vi "MB Ethernet Master Query.vi"(4 "Timeout":i32=5000, 6 "MBAP Header":cluster{"Transaction ID":u16, "Unit ID":u8}, 7 "Modbus Data Unit In":T2={"Function Code"=1, "Data"=[]} {"Function Code" items=["Read Coils"=1, "Read Discrete Inputs"=2, "Read Holding Registers"=3, "Read Input Registers"=4, "Write Single Coil"=5, "Write Single Register"=6, "Read Exception Status"=7, "Write Multiple Coils"=15, "Write Multiple Registers"=16]; "Data" format="%.0x"}, 8 "error in (no error)":errorcluster, 9 "Use MODBUS Data Unit?":bool, 10 "Modbus Command":T1={"Function Code"=1, "Starting Address"=0, "Quantity"=0, "Data"=[], "Discrete"=[]} {"Function Code" items=["Read Coils"=1, "Read Discrete Inputs"=2, "Read Holding Registers"=3, "Read Input Registers"=4, "Write Single Coil"=5, "Write Single Register"=6, "Read Exception Status"=7, "Write Multiple Coils"=15, "Write Multiple Registers"=16]}, 11 "TCP Connection Refnum in":refnum<k5>) -> (0 "error out":errorcluster, 1 "Exception Code":u8 format="%.0x", 2 "Registers":cluster{"Registers":u16[], "Discrete":bool[]}, 3 "TCP Connection Refnum (dup)":refnum<k5>, 5 "Modbus Data Unit Out":T2={"Function Code"=1, "Data"=[]} {"Function Code" items=["Read Coils"=1, "Read Discrete Inputs"=2, "Read Holding Registers"=3, "Read Input Registers"=4, "Write Single Coil"=5, "Write Single Register"=6, "Read Exception Status"=7, "Write Multiple Coils"=15, "Write Multiple Registers"=16]; "Data" format="%.0x"})   [LabVIEW 2023, in "Voegtlin_NI_SMART_Modbus_Drivers.lvlib"]
uses:
  Voegtlin_NI_SMART_Modbus_Drivers.lvlib
  MB Modbus Data Unit.ctl
  MB Modbus Command.ctl
panel:
  # "VI Name: MB Ethernet Master Query.vi\nPurpose: Performs a Modbus TCP query."
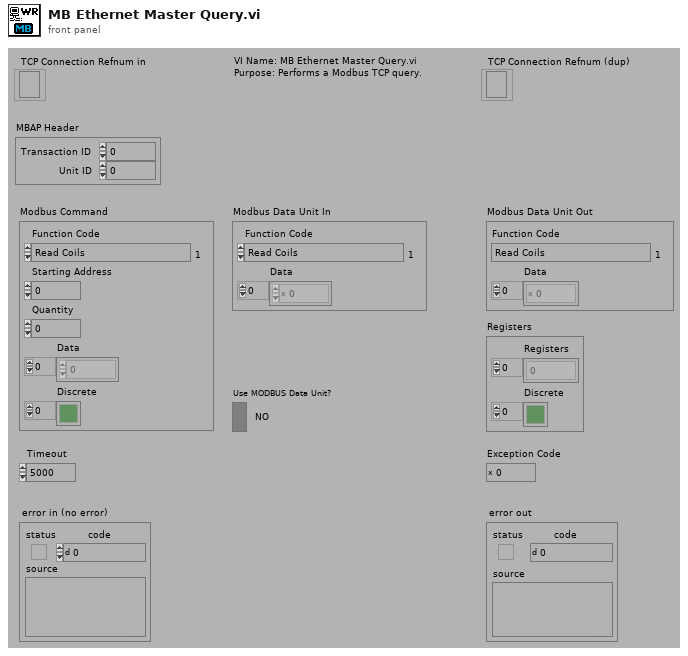
[diagram p1: front panel]
types:
  T1 = typedef "Voegtlin_NI_SMART_Modbus_Drivers.lvlib/MB Modbus Command.ctl" = cluster{"Function Code":u8, "Starting Address":u16, "Quantity":u16, "Data":u16[], "Discrete":bool[]}
  T2 = typedef "Voegtlin_NI_SMART_Modbus_Drivers.lvlib/MB Modbus Data Unit.ctl" = cluster{"Function Code":u8, "Data":u8[]}
  T3 = cluster{"Transaction ID":u16, "Protocol ID":u16, "Length":u16, "Unit ID":u8}
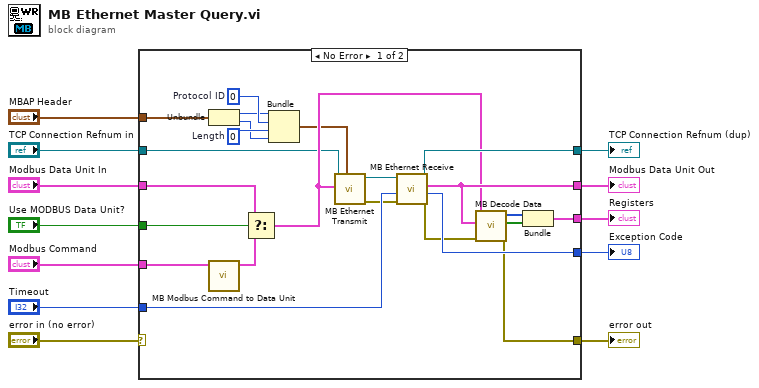
[diagram p0: block diagram]
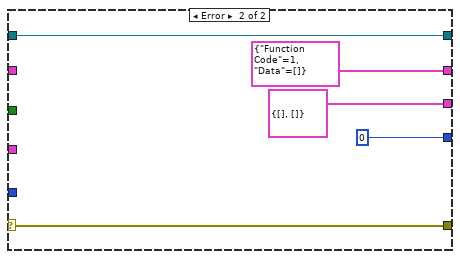
[diagram p2: hidden frame]
diagram:
  n1 = case shown="No Error" "error in (no error)" {
    selector: "error in (no error)" -> [_ w36]
    tunnel: [w29 T2 {"Function Code"=1, "Data"=[]} ("MODBUS Data Unit")] -> w5
    tunnel: [w33 u8 0 ("Exception Code")] -> w12
    tunnel: [w27 w36] -> w3
    tunnel: "TCP Connection Refnum in" -> [w19 w40]
    tunnel: "Timeout" -> [w35 _]
    tunnel: [w34 w40] -> w9
    tunnel: "Modbus Data Unit In" -> [w32 _]
    tunnel: "Use MODBUS Data Unit?" -> [w31 _]
    tunnel: "Modbus Command" -> [w30 _]
    tunnel: [w28 cluster{"Registers":u16[], "Discrete":bool[]} {"Registers"=[], "Discrete"=[]}] -> w4
    tunnel: "MBAP Header" -> [w17 _]
    frame No Error {
      w14 = u16 0  # Length
      w16 = u16 0  # Protocol ID
      n2 = Unbundle(w17) -> ("Transaction ID"=w15:u16, "Unit ID"=w13:u8)
      n3 = call "MB Modbus Command to Data Unit.vi"("Modbus Command"=w30) -> ("Modbus Data Unit"=w26:T2)  [unwired: 10 out]
      n4 = Select(t=w32, s=w31, f=w26) -> (s? t:f=w22:T2)
      n5 = Bundle("Transaction ID"=w15, "Protocol ID"=w16, "Length"=w14, "Unit ID"=w13) -> (w18:T3)  [unwired: 1 out]
      n6 = call "MB Ethernet Transmit.vi"("MBAP Header"=w18, "Modbus Data Unit"=w22, "TCP Connection Refnum in"=w19) -> ("error out"=w20:errorcluster, "TCP Connection Refnum (dup)"=w21:refnum<k5>)  [unwired: 2 in, 5 out]
      n7 = call "MB Ethernet Receive.vi"("error in (no error)"=w20, "Timeout"=w35, "Connection ID"=w21) -> ("error out"=w25:errorcluster, "Exception Code"=w33:u8, "Modbus Data Unit"=w29:T2, "Connection ID (dup)"=w34:refnum<k5>)  [unwired: 5 out]
      n8 = call "MB Decode Data.vi"("error in (no error)"=w25, "Response MDU"=w29, "Request MDU"=w22) -> ("error out"=w27:errorcluster, "Discrete"=w23:bool[], "Registers"=w24:u16[])  [unwired: 6 out]
      n9 = Bundle("Registers"=w24, "Discrete"=w23) -> (w28:cluster{"Registers":u16[], "Discrete":bool[]})  [unwired: 1 out]
    }
    frame Error {
    }
  }
  "error out" <- w3
  "Exception Code" <- w12
  "TCP Connection Refnum (dup)" <- w9
  "Modbus Data Unit Out" <- w5
  "Registers" <- w4
